vi "receive_data.vi"(8 "error in (no error)":errorcluster, 11 "TCP Network Connection in":refnum<k5>) -> (0 "error out":errorcluster, 1 "XY Graph":cluster{dbl[], dbl[]}(graph), 2 "Valori asse y":dbl[](array[numeric]), 3 "TCP Network Connection out":refnum<k5>, 4 "Valori asse x":dbl[](array[numeric]), 5 "Frequenza -3dB":dbl)   [LabVIEW 2021]
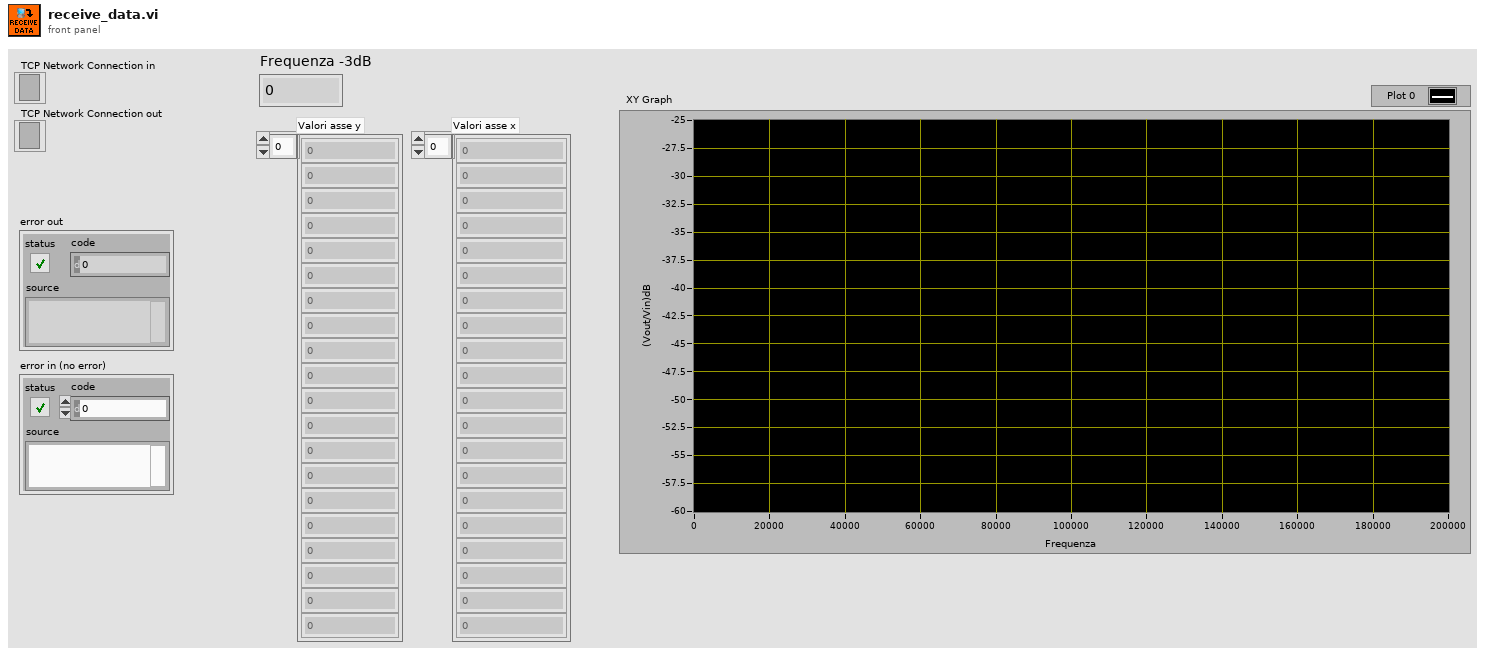
[diagram p1: front panel]
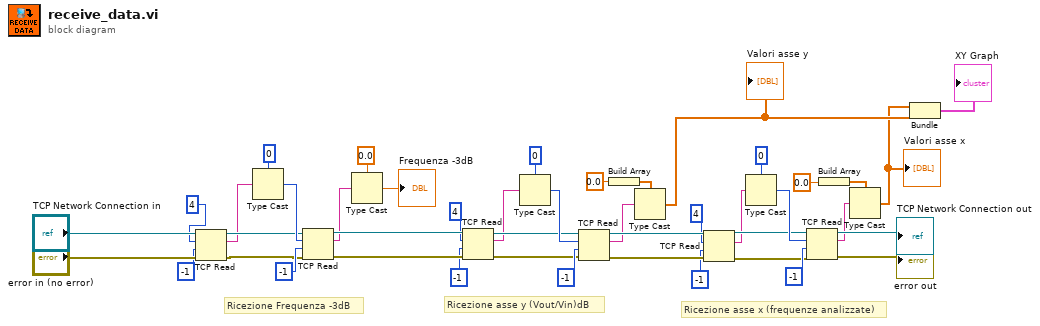
[diagram p0: block diagram]
diagram:
  # "Ricezione asse x (frequenze analizzate)"
  # "Ricezione asse y (Vout/Vin)dB"
  # "Ricezione Frequenza -3dB"
  n1 = TCP Read(connection ID="TCP Network Connection in", bytes to read=4, error in (no error)="error in (no error)", 9:-1 ("timeout ms (25000)")) -> (connection ID out=w14:refnum<k5>, data out=w12:string, error out=w15:errorcluster)  [unwired: 1 in]
  n2 = Type Cast(type=0, x=w12) -> (*(type *) &x=w18:i32)
  n3 = TCP Read(connection ID=w14, bytes to read=w18, error in (no error)=w15, 9:-1 ("timeout ms (25000)")) -> (connection ID out=w35:refnum<k5>, data out=w9:string, error out=w34:errorcluster)  [unwired: 1 in]
  n4 = Type Cast(type=0.0, x=w9) -> (*(type *) &x=→"Frequenza -3dB":dbl)
  n5 = TCP Read(connection ID=w35, bytes to read=4, error in (no error)=w34, 9:-1 ("timeout ms (25000)")) -> (connection ID out=w3:refnum<k5>, data out=w1:string, error out=w4:errorcluster)  [unwired: 1 in]
  n6 = Type Cast(type=0 ("timeout ms (25000)"), x=w1) -> (*(type *) &x=w39:i32)
  n7 = TCP Read(connection ID=w3, bytes to read=w39, error in (no error)=w4, 9:-1 ("timeout ms (25000)")) -> (connection ID out=w33:refnum<k5>, data out=w6:string, error out=w32:errorcluster)  [unwired: 1 in]
  n8 = Build Array(0.0) -> (w7:dbl[])
  n9 = Type Cast(type=w7, x=w6) -> (*(type *) &x=w42:dbl[])
  "Valori asse y" <- w42
  n10 = TCP Read(connection ID=w33, bytes to read=4, error in (no error)=w32, 9:-1 ("timeout ms (25000)")) -> (connection ID out=w23:refnum<k5>, data out=w21:string, error out=w24:errorcluster)  [unwired: 1 in]
  n11 = Type Cast(type=0 ("timeout ms (25000)"), x=w21) -> (*(type *) &x=w40:i32)
  n12 = TCP Read(connection ID=w23, bytes to read=w40, error in (no error)=w24, 9:-1 ("timeout ms (25000)")) -> (connection ID out=→"TCP Network Connection out":refnum<k5>, data out=w26:string, error out=→"error out":errorcluster)  [unwired: 1 in]
  n13 = Build Array(0.0) -> (w27:dbl[])
  n14 = Type Cast(type=w27, x=w26) -> (*(type *) &x=w41:dbl[])
  "Valori asse x" <- w41
  n15 = Bundle(w41, w42) -> (→"XY Graph":cluster{dbl[], dbl[]})  [unwired: 1 in]
